vi "Map Range.vi"(8 "error in (no error)":errorcluster, 10 "Range":refnum<class "Range.lvclass">, 11 "Range Map in":refnum<class "Range Map.lvclass">) -> (0 "error out":errorcluster, 2 "Ranges":refnum<class "Range.lvclass">[](array[class]), 3 "Range Map out":refnum<class "Range Map.lvclass">)   [LabVIEW 2020, in "Range Map.lvclass"]
uses:
  Range Map.lvclass
  Range/Range.lvclass
  Range Map.lvclass/Range Map.ctl
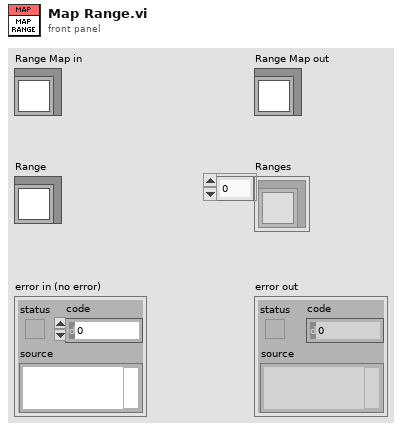
[diagram p1: front panel]
types:
  T1 = cluster{"Source":refnum<class "Range.lvclass">, "Destination":refnum<class "Range.lvclass">}[]
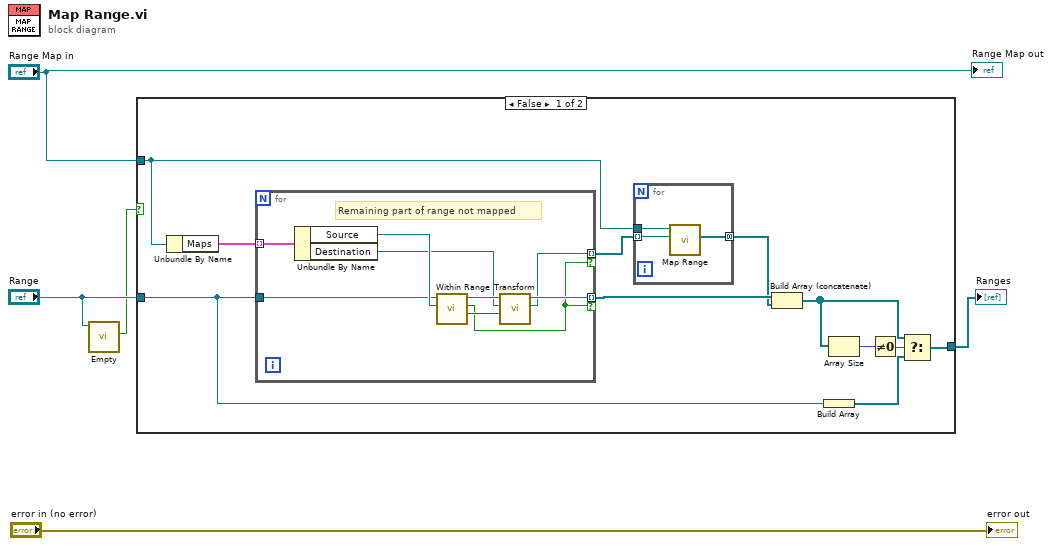
[diagram p0: block diagram]
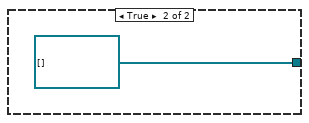
[diagram p2: hidden frame]
diagram:
  n1 = call "Empty"("Range in"="Range") -> ("Boolean"=w1:bool)  [unwired: 8 in, 2 out]
  n2 = case shown="False" w1 {
    tunnel: [w11 refnum<class "Range.lvclass">[] []] -> w4
    tunnel: "Range Map in" -> [w10 _]
    tunnel: "Range" -> [w8 _]
    frame False {
      n3 = Unbundle By Name(w10) -> ("Maps"=w16:T1)
      n4 = for {
        tunnel: w16 -> [w28] mode=indexing
        tunnel: w8 -> [w26]
        tunnel: [w23] -> w12 mode=indexing if=w20
        tunnel: [w21] -> w7 mode=indexing if=w20
        # "Remaining part of range not mapped"
        n5 = Unbundle By Name(w28) -> ("Source"=w27:refnum<class "Range.lvclass">, "Destination"=w24:refnum<class "Range.lvclass">)
        n6 = call "Within Range.vi"("Range to compare to"=w27, "Range in"=w26) -> ("Offset"=w22:u64, "In Range?"=w20:bool, "Range out"=w25:refnum<class "Range.lvclass">)  [unwired: 6 in, 1 out]
        n7 = call "Transform.vi"("Offset"=w22, "Transformation Map"=w24, "Range in"=w25) -> ("Remainder"=w21:refnum<class "Range.lvclass">, "Range out"=w23:refnum<class "Range.lvclass">)  [unwired: 6 in, 1 out]
      }
      n8 = for {
        tunnel: w10 -> [w19]
        tunnel: w7 -> [w18] mode=indexing
        tunnel: [w17] -> w6 mode=concatenating
        n9 = call "Map Range.vi"("Range"=w18, "Range Map in"=w19) -> ("Ranges"=w17:refnum<class "Range.lvclass">[])  [unwired: 7 in, 2 out]
      }
      n10 = Build Array (concatenate)(w12, w6) -> (w9:refnum<class "Range.lvclass">[])
      n11 = Build Array(w8) -> (w13:refnum<class "Range.lvclass">[])
      n12 = Array Size(array=w9) -> (size(s)=w15:i32)
      n13 = Not Equal To 0?(x=w15) -> (x != 0?=w14:bool)
      n14 = Select(t=w9, s=w14, f=w13) -> (s? t:f=w11:refnum<class "Range.lvclass">[])
    }
    frame True {
    }
  }
  "Ranges" <- w4
  "error out" <- "error in (no error)"
  "Range Map out" <- "Range Map in"
